vi "Module Loop.vi"(8 "error in (no error)":errorcluster, 11 "ValveControlModule in":refnum<class "DigitalControlModule.lvclass">) -> (0 "error out":errorcluster, 3 "ValveControlModule out":refnum<class "DigitalControlModule.lvclass">)   [LabVIEW 2023, in "VolatusControl.lvlib" / "DigitalControlModule.lvclass"]
uses:
  DigitalControlModule.lvclass
  DigitalControlModule.lvclass/DigitalControlModule.ctl
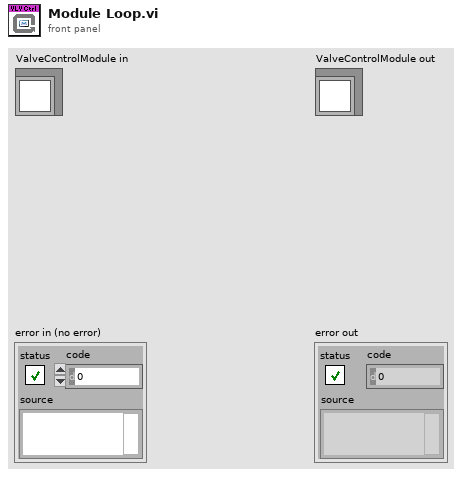
[diagram p1: front panel]
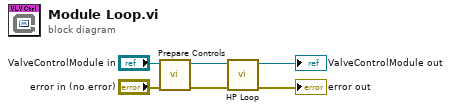
[diagram p0: block diagram]
diagram:
  n1 = call "Prepare Controls.vi"("error in (no error)"="error in (no error)", "ValveControlModule in"="ValveControlModule in") -> ("error out"=w4:errorcluster, "ValveControlModule out"=w2:refnum<class "DigitalControlModule.lvclass">)  [unwired: 8 in]
  n2 = call "HP Loop.vi"("error in (no error)"=w4, "ValveControlModule in"=w2) -> ("error out"=→"error out":errorcluster, "ValveControlModule out"=→"ValveControlModule out":refnum<class "DigitalControlModule.lvclass">)  [unwired: 8 in]
